vi "数字麦克风信号解析.vi"() -> ()   [LabVIEW 2024]
panel:
  out "文本":string
  out "波形图":i32[](graph)
  in  "路径":path=path "D:/Labviewworks/数字麦克风信号解析/采集数据文件/6060.log"
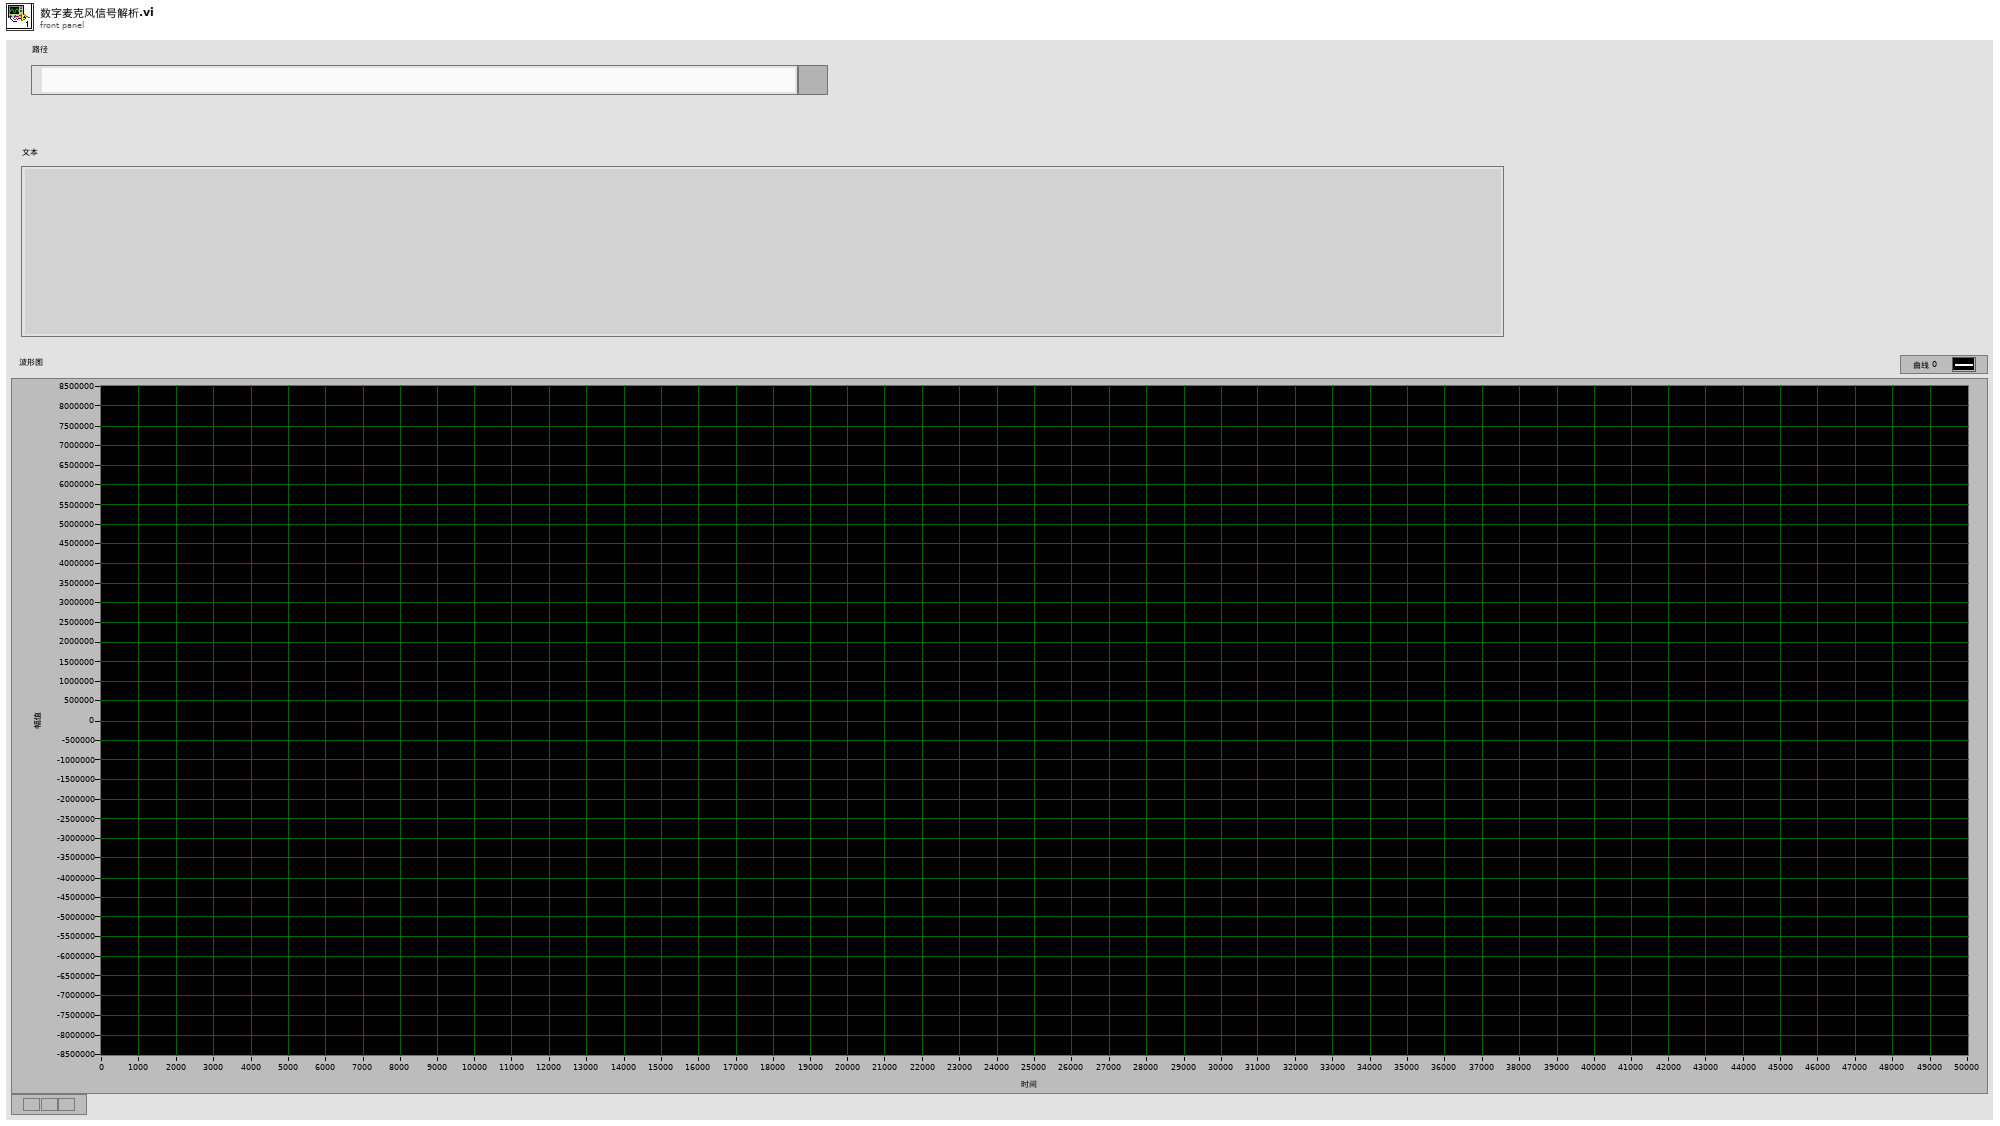
[diagram p1: front panel]
types:
  T1 = enum16{"open", "replace", "create", "open or create", "replace or create", "replace or create with confirmation"}
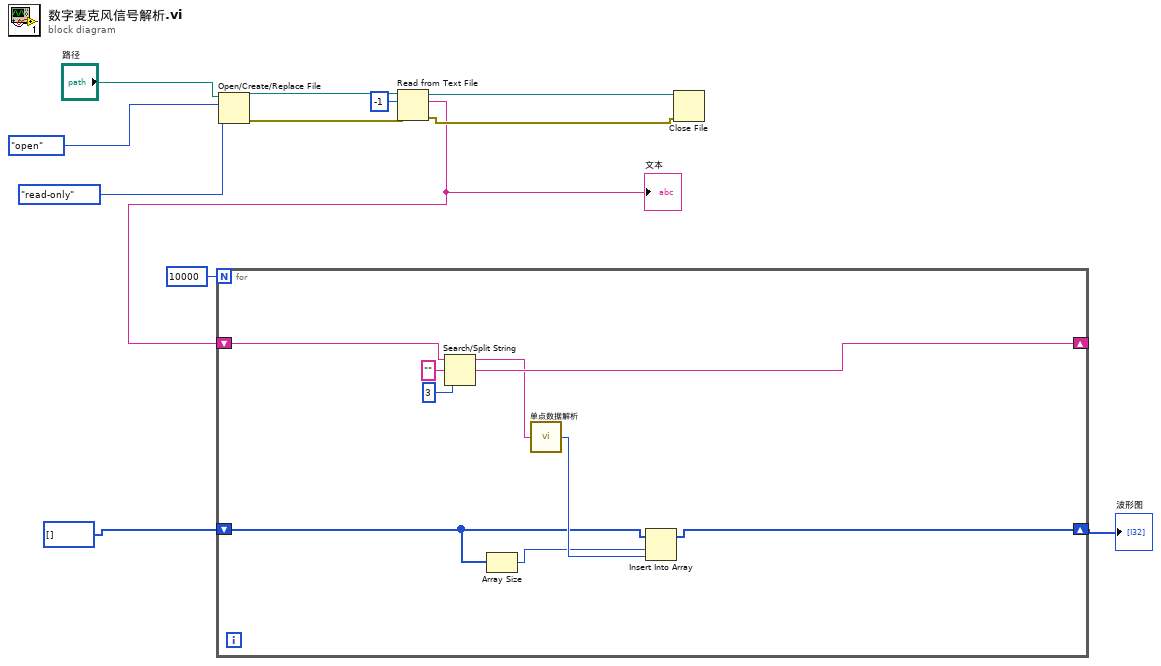
[diagram p0: block diagram]
diagram:
  n1 = Open/Create/Replace File(file path (use dialog)="路径", operation (0:open)=T1."open" ("操作(0:open)"), access (0:read/write)=enum16{"read/write", "read-only", "write-only"}."read-only" ("权限(0:read/write)")) -> (refnum out=w9:refnum<file>, error out=w8:errorcluster)  [unwired: 3 in, 1 out]
  n2 = Read from Text File(file (use dialog)=w9, count=-1 ("计数"), error in=w8) -> (refnum out=w7:refnum<file>, text=w4:string, error out=w6:errorcluster)  [unwired: 1 in, 1 out]
  "文本" <- w4
  n3 = for {
    N: 10000 -> [_]
    shift-right: [w18] -> _
    shift-left: w4 -> [w21]
    shift-right: [w13] -> w1
    shift-left: i32[] [] -> [w15]
    n4 = Search/Split String(string=w21, search string/char (-)="" ("搜索字符串/字符(-)"), offset (0)=3 ("偏移量(0)")) -> (substring before match=w17:string, match + rest of string=w18:string)  [unwired: 1 out]
    n5 = Array Size(array=w15) -> (size(s)=w14:i32)
    n6 = call "单点数据解析.vi"("字符串"=w17) -> ("*(类型 *) &x"=w16:i32)  [unwired: 4 in]
    n7 = Insert Into Array(array=w15, index=w14, new element=w16) -> (w13:i32[])
  }
  "波形图" <- w1
  n8 = Close File(refnum=w7, error in=w6) -> ()  [unwired: 2 out]
